vi "GernateViDoc.vi"() -> ()   [LabVIEW 2020]
panel:
  out "error out":errorcluster
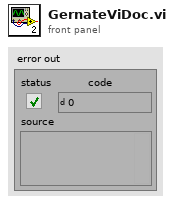
[diagram p1: front panel]
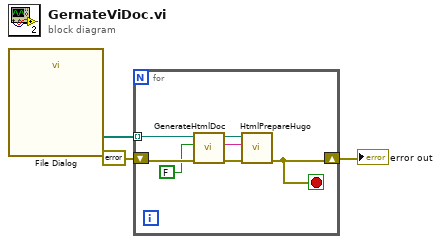
[diagram p0: block diagram]
diagram:
  n1 = call "File Dialog"() -> ("selected paths"=w3:path[])  [unwired: 12 in, 3 out]
  n2 = for {
    shift-right: [w6] -> w2
    shift-left: errorcluster {"status"=FALSE, "code"=0, "source"=""} ("error out") -> [w7]
    tunnel: w3 -> [w5] mode=indexing
    stop <- w6 stop-if-true
    n3 = call "GenerateHtmlDoc.vi"("error in"=w7, "Clear"=FALSE, "Vi"=w5) -> ("error out"=w10:errorcluster, "VI Description"=w8:string, "Html Path"=w9:path)  [unwired: 6 in]
    n4 = call "HtmlPrepareHugo.vi"("error in"=w10, "ViDescr"=w8, "Html Path"=w9) -> ("error out"=w6:errorcluster)  [unwired: 8 in]
  }
  "error out" <- w2
